vi "create junit report.vi"(8 "Error In (No Error)":errorcluster, 10 "junit report file path":path, 11 "test results":T3) -> (0 "Error Out":errorcluster)   [LabVIEW 2013]
uses:
  <vilib>/utf/dialogs/utf_testsuite_report_sortby.ctl
  <vilib>/utf/results/utf_report_summary.ctl
  <vilib>/utf/common/utf_test_result_overall.ctl
  <vilib>/utf/common/utf_test_result_testfile.ctl
  <vilib>/utf/common/utf_test_result_testcase.ctl
  <vilib>/utf/common/utf_test_result.ctl
  <vilib>/utf/common/utf_test_result_troll_new.ctl
  <vilib>/utf/common/utf_vector_result.ctl
  <vilib>/utf/common/utf_test_result_failure.ctl
  <vilib>/utf/common/utf_test_comparison_operators.ctl
  <vilib>/utf/common/utf_vi_tag.ctl
  <vilib>/utf/common/utf_test_result_input_data.ctl
  <vilib>/utf/common/utf_code_coverage.ctl
  <vilib>/utf/common/utf_error_data.ctl
  <vilib>/utf/common/utf_error_type.ctl
  <vilib>/utf/common/utf_subvi_info.ctl
  <vilib>/utf/dialogs/utf_testsuite_report_settings.ctl
  <vilib>/NI/JUnit Results API/Controls/Test Suites Attribute Values.ctl
  <vilib>/NI/JUnit Results API/Controls/Test Case Attributes.ctl
  <vilib>/NI/JUnit Results API/Controls/Outcome Attributes.ctl
  <vilib>/xml/Close Reference(Node).vi
  <vilib>/NI/JUnit Results API/JUnit API.lvlib
  <vilib>/xml/NI_XML.lvlib
  <vilib>/utf/NI_UnitTestFramework.lvlib
panel:
  in  "Report config":T1={"View Report ATML"=FALSE, "Create text report"=FALSE, "TEXT Sort by"=0, "ASCII report Path (*.txt)"=path "", "Create html report"=FALSE, "HTML report Path (*.html)"=path "", "Create atml report"=FALSE, "ATML report Path (*.xml)"=path "", "Summary Data"=FALSE, "Failed Tests"=TRUE, "Failed Tests Details"=TRUE, "Passed Tests"=TRUE, "Passed Tests Details"=TRUE, "Skipped Tests"=FALSE, "Errors"=FALSE, "Stylesheet file (*.css)"=path "", "Use stylesheet"=TRUE, "View Report HTML"=FALSE, "View Report TXT"=FALSE, "Errors Detail"=FALSE, "calculate project code coverage"=FALSE} {"TEXT Sort by" items=["VI name", "Test name"]}
  out "summary":T17
  in  "Sort by":T2=1 items=["VI name", "Test name"]
  # "Report Settings"
  # "Sort by"
  # "Report Content"
  # "HTML Stylesheet"
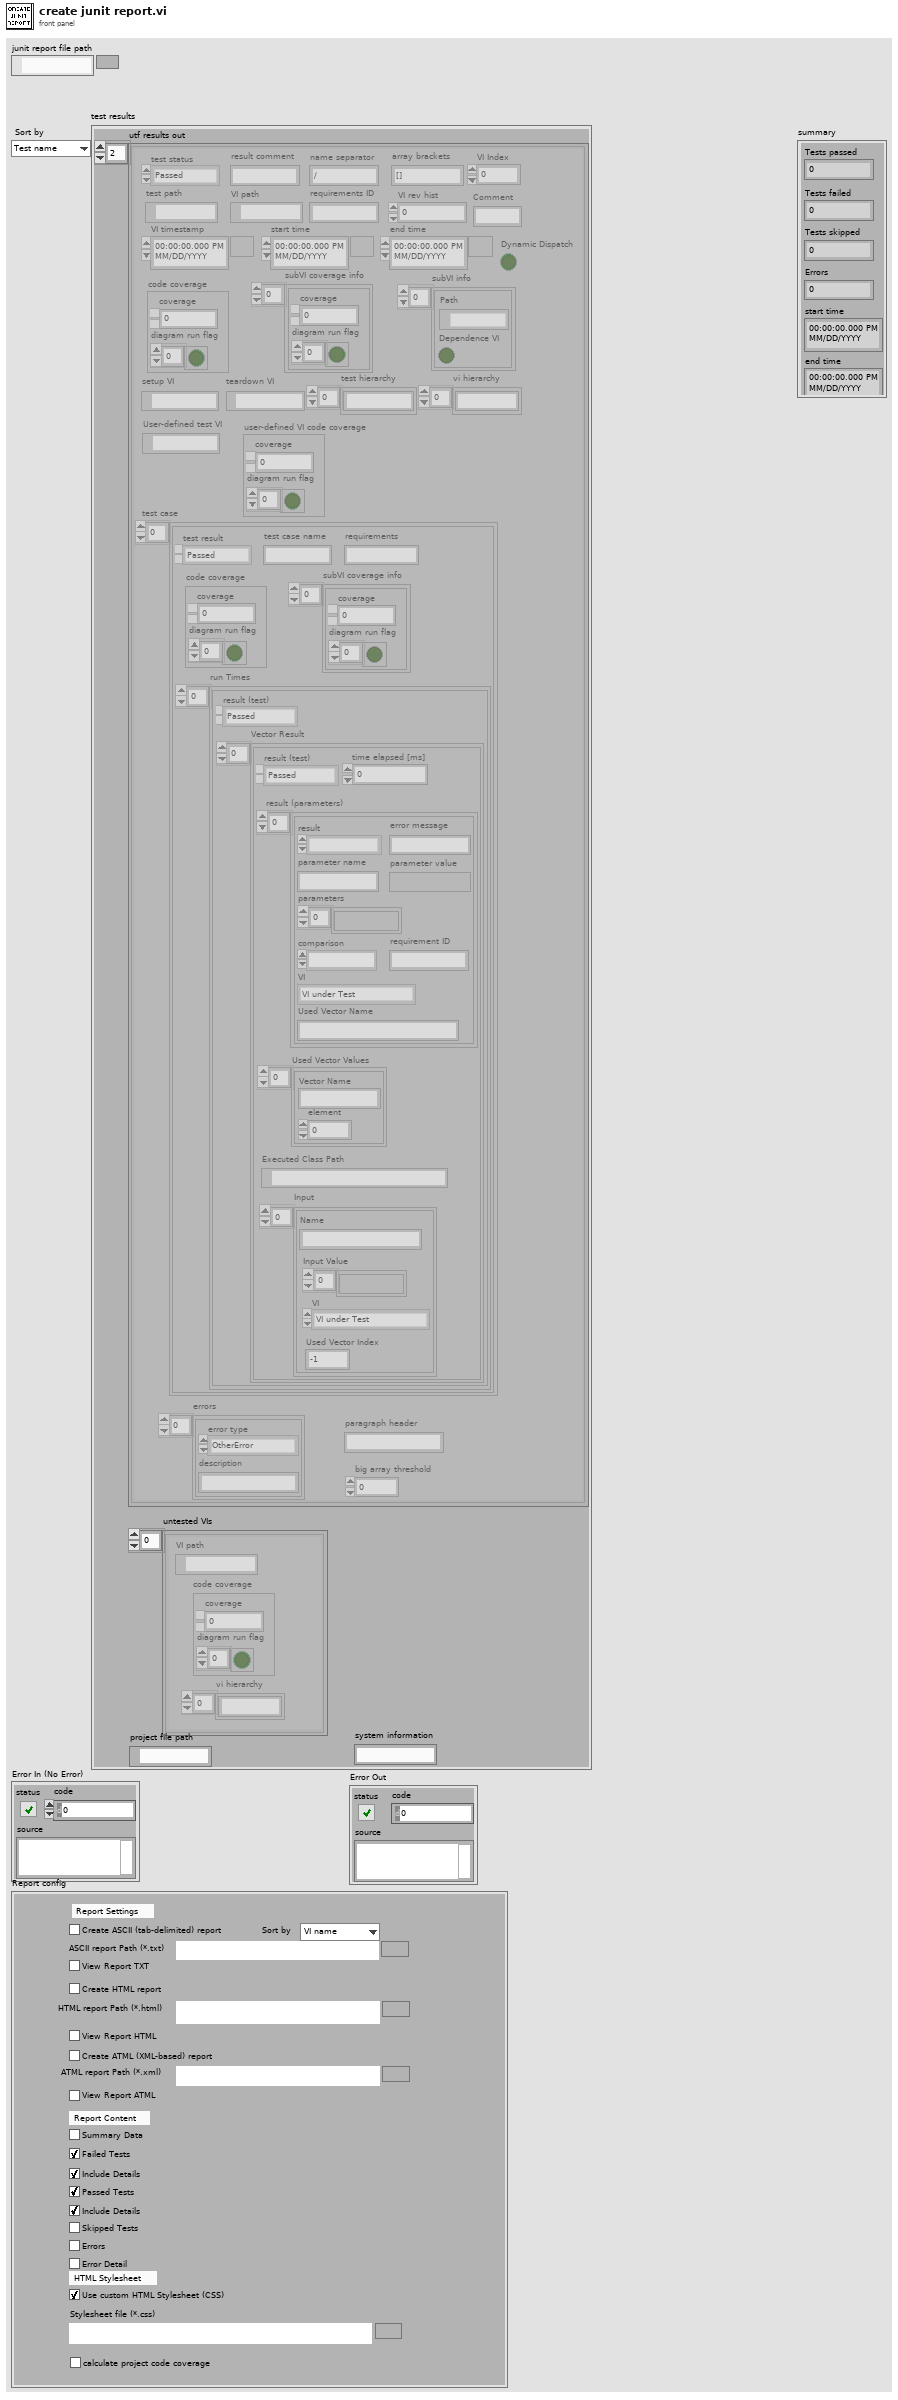
[diagram p1: front panel]
types:
  T1 = typedef "NI_UnitTestFramework.lvlib/utf_testsuite_report_settings.ctl" = cluster{"View Report ATML":bool, "Create text report":bool, "TEXT Sort by":T2, "ASCII report Path (*.txt)":path, "Create html report":bool, "HTML report Path (*.html)":path, "Create atml report":bool, "ATML report Path (*.xml)":path, "Summary Data":bool, "Failed Tests":bool, "Failed Tests Details":bool, "Passed Tests":bool, "Passed Tests Details":bool, "Skipped Tests":bool, "Errors":bool, "Stylesheet file (*.css)":path, "Use stylesheet":bool, "View Report HTML":bool, "View Report TXT":bool, "Errors Detail":bool, "calculate project code coverage":bool}
  T2 = typedef "NI_UnitTestFramework.lvlib/utf_testsuite_report_sortby.ctl" = u16
  T3 = typedef "NI_UnitTestFramework.lvlib/utf_test_result_overall.ctl" = cluster{"utf results out":T4[], "untested VIs":cluster{"VI path":path, "code coverage":T13, "vi hierarchy":string[]}[], "project file path":path, "system information":string}
  T4 = typedef "NI_UnitTestFramework.lvlib/utf_test_result_testfile.ctl" = cluster{"test case":T5[], "test status":T6, "test path":path, "setup VI":path, "teardown VI":path, "code coverage":T13, "start time":timestamp, "end time":timestamp, "test hierarchy":string[], "VI path":path, "VI timestamp":timestamp, "VI rev hist":i32, "requirements ID":string, "array brackets":string, "name separator":string, "errors":T14[], "paragraph header":string, "result comment":string, "vi hierarchy":string[], "subVI coverage info":T13[], "subVI info":T16[], "big array threshold":u32, "VI Index":i32, "Comment":string, "Dynamic Dispatch":bool, "User-defined test VI":path, "user-defined VI code coverage":T13}
  T5 = typedef "NI_UnitTestFramework.lvlib/utf_test_result_testcase.ctl" = cluster{"test result":T6, "run Times":T7[], "test case name":string, "requirements":string, "code coverage":T13, "subVI coverage info":T13[]}
  T6 = typedef "NI_UnitTestFramework.lvlib/utf_test_result.ctl" = enum16{"Passed", "Failed", "Error", "Skipped", "Not Processed"}
  T7 = typedef "NI_UnitTestFramework.lvlib/utf_test_result_troll_new.ctl" = cluster{"result (test)":T6, "Vector Result":T8[]}
  T8 = typedef "NI_UnitTestFramework.lvlib/utf_vector_result.ctl" = cluster{"time elapsed [ms]":u32, "result (test)":T6, "result (parameters)":T9[], "Used Vector Values":cluster{"Vector Name":string, "element":i32}[], "Executed Class Path":path, "Input":T12[]}
  T9 = typedef "NI_UnitTestFramework.lvlib/utf_test_result_failure.ctl" = cluster{"result":T6, "error message":string, "parameter name":string, "parameter value":variant, "parameters":variant[], "comparison":T10, "requirement ID":string, "VI":T11, "Used Vector Name":string}
  T10 = typedef "NI_UnitTestFramework.lvlib/utf_test_comparison_operators.ctl" = enum16{"=", "!=", ">", ">=", "<", "<=", "range", "symmetric tolerance", "asymmetric tolerance", "string contains", "string not contain", "array size", "string length", "array range", "by element", "array range (limit array)", "user-defined", "array contains", "array not contain", "vector length", "= (elm)", "!= (elm)", "= (case insensitive)", "!= (case insensitive)"}
  T11 = typedef "NI_UnitTestFramework.lvlib/utf_vi_tag.ctl" = enum16{"Setup VI", "VI under Test", "Teardown VI"}
  T12 = typedef "NI_UnitTestFramework.lvlib/utf_test_result_input_data.ctl" = cluster{"Name":string, "Input Value":variant[], "VI":T11, "Used Vector Index":i32}
  T13 = typedef "NI_UnitTestFramework.lvlib/utf_code_coverage.ctl" = cluster{"coverage":dbl, "diagram run flag":bool[]}
  T14 = typedef "NI_UnitTestFramework.lvlib/utf_error_data.ctl" = cluster{"error type":T15, "description":string}
  T15 = typedef "NI_UnitTestFramework.lvlib/utf_error_type.ctl" = enum16{"TestFileError", "VIError", "SetupVIError", "TearDownVIError", "OtherError"}
  T16 = typedef "NI_UnitTestFramework.lvlib/utf_subvi_info.ctl" = cluster{"Path":path, "Dependence VI":bool}
  T17 = typedef "NI_UnitTestFramework.lvlib/utf_report_summary.ctl" = cluster{"Tests passed":i32, "Tests failed":i32, "Tests skipped":i32, "Errors":i32, "start time":timestamp, "end time":timestamp}
  T18 = typedef "JUnit API.lvlib/Test Suites Attribute Values.ctl" = cluster{"name":string, "time":dbl, "tests":i32, "failures":i32, "disabled":i32, "errors":i32}
  T19 = typedef "JUnit API.lvlib/Test Case Attributes.ctl" = cluster{"name":string, "assertions":i32, "time":dbl, "timestamp":dbl, "classname":string, "status":string, "class":string, "file":string, "line":string, "log":string, "group":string, "url":string}
  T20 = typedef "JUnit API.lvlib/Outcome Attributes.ctl" = cluster{"message":string, "type":string}
  T21 = typedef "JUnit API.lvlib/Test Suite Attribute Values.ctl" = cluster{"name":string, "tests":i32, "failures":i32, "errors":i32, "time":dbl, "disabled":i32, "skipped":i32, "skips":i32, "timestamp":dbl, "hostname":string, "id":string, "package":string, "assertions":i32, "file":string, "skip":string, "log":string, "url":string}
  T22 = typedef "NI_UnitTestFramework.lvlib/utf_test_properties.ctl" = cluster{"Test File Header":T23, "Test Values":T27[], "Setup Teardown Info":T31, "Setup Values":T27[], "Teardown Values":T27[], "Vector Info":cluster{"included vector files":path[], "vector array":T34[], "included and inherited vector files":path[]}}
  T23 = typedef "NI_UnitTestFramework.lvlib/utf_test_file_header.ctl" = cluster{"Test Name":string, "Comment":string, "VI Under Test":path, "Library":path, "Priority":u32, "Test Vector Execution":T24, "Array Brackets":string, "Requirements ID":string, "Skip for project window":bool, "Skip for palette VI":bool, "Repetitions":u32, "Set time-out":bool, "Time-out":u32, "Check Code Coverage":bool, "Minimum Code Coverage":u32, "User-defined Test":bool, "Name Separator":string, "User-defined Test VI":path, "Precision":u8, "Creation Type":T25, "Decimal separator":string, "Big Array Threshold":u32, "Save control names in normal format":bool, "Capture Input Value":bool, "Capture Output Value":bool, "Version":string, "Set automatic error handling":T26, "Remove breakpoints":bool}
  T24 = typedef "NI_UnitTestFramework.lvlib/utf_test_processing.ctl" = enum16{"None", "Linear", "Permutations"}
  T25 = typedef "NI_UnitTestFramework.lvlib/utf_test_creation_type.ctl" = enum16{"Include controls and indicators from connector pane", "Include controls and indicators from front panel", "Include controls and indicators from front panel as both input and output"}
  T26 = typedef "NI_UnitTestFramework.lvlib/utf_set_automatic_error_handling.ctl" = enum16{"As is", "Enable", "Disable"}
  T27 = typedef "NI_UnitTestFramework.lvlib/utf_test_values_cluster.ctl" = cluster{"Input Values Array":T28[], "Expected Values Array":T30[], "Test Case Name":string, "Test Case Comment":string}
  T28 = typedef "NI_UnitTestFramework.lvlib/utf_test_input_values.ctl" = cluster{"Name":string, "Data type":T29, "Input Value":variant[], "Default Flag":bool, "Requirements ID":string, "Array Type":i8, "Typedef Flag":bool, "Setup Flag":bool, "Terminal":string, "Global Variable":bool, "type information":variant, "Shared Variable":bool, "Use Vector":bool, "Vector Name":string, "Index":u8}
  T29 = typedef "VariantType.lvlib/Type.ctl" = enum8{"Invalid Type", "Void", "I8", "I16", "I32", "I64", "U8", "U16", "U32", "U64", "Single Float", "Double Float", "Extended Float", "Single Complex", "Double Complex", "Extended Complex", "Enum U8", "Enum U16", "Enum U32", "Enum U64", "Single Float With Unit", "Double Float With Unit", "Extended Float With Unit", "Single Complex with Unit", "Double Complex with Unit", "Extended Complex with Unit", "Boolean", "String", "Path", "Picture", "Tag", "Array", "Cluster", "Variant", "LV Variant", "Waveform", "Timestamp", "Digital Waveform", "Digital Data", "ExpressData", "Refnum", "External Data", "VI", "Poly VI", "LabVIEW Class Instance", "Fixed Point"}
  T30 = typedef "NI_UnitTestFramework.lvlib/utf_test_expected_values.ctl" = cluster{"Name":string, "Data type":T29, "Expected value":variant, "Check flag":bool, "Typedef Flag":bool, "Comparison":T10, "User-defined Comparison VI":path, "Requirements ID":string, "Array Type":i8, "by element":dbl, "Teardown Flag":bool, "Terminal":string, "Global Variable":bool, "type information":variant, "Shared Variable":bool, "By Element":bool, "Use Vector":bool, "Vector Name":string}
  T31 = typedef "NI_UnitTestFramework.lvlib/utf_setup_teardown_info.ctl" = cluster{"Setup VI":path, "Teardown VI":path, "Setup Data":T32[], "Teardown Data":T33[]}
  T32 = typedef "NI_UnitTestFramework.lvlib/utf_setup_info.ctl" = cluster{"Terminal":string, "Input":string}
  T33 = typedef "NI_UnitTestFramework.lvlib/utf_teardown_info.ctl" = cluster{"Terminal":string, "Output":string}
  T34 = typedef "NI_UnitTestFramework.lvlib/utf_vector_info.ctl" = cluster{"requirement ID":string, "file path":path, "Data type":T29, "append":string, "size":u64, "name":string, "vector edit type":enum16{"sequence", "linear"}, "values":variant[], "qualify name":string}
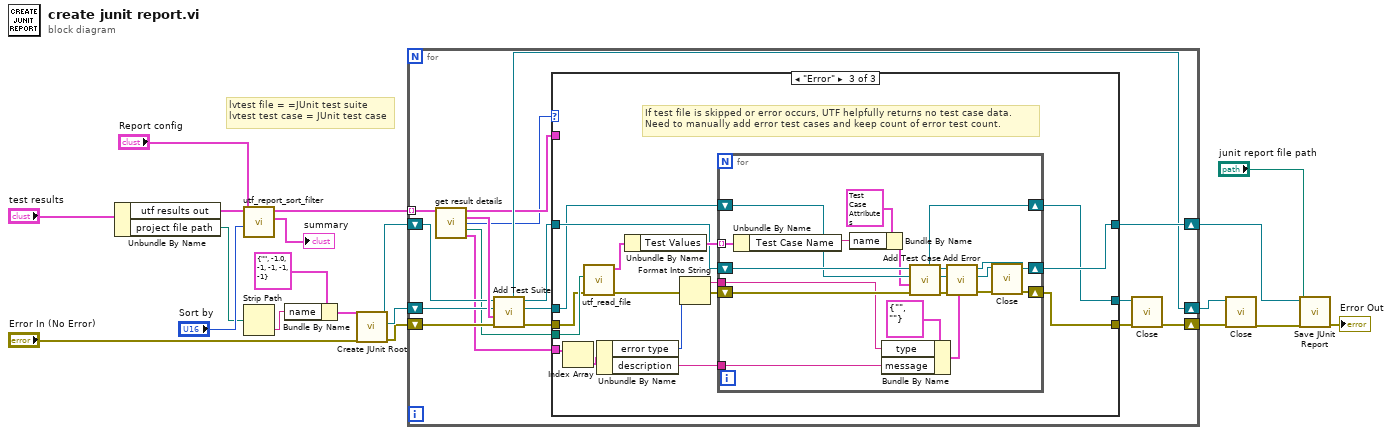
[diagram p0: block diagram]
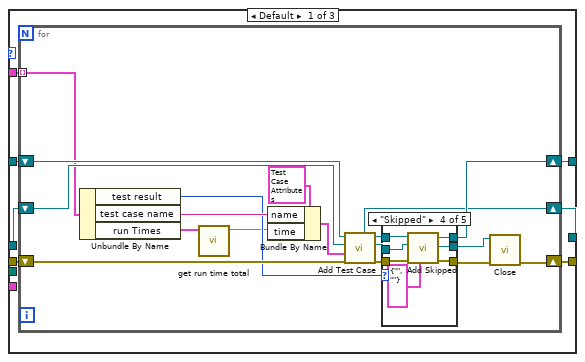
[diagram p2: hidden frame]
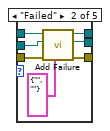
[diagram p4: hidden frame]
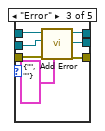
[diagram p5: hidden frame]
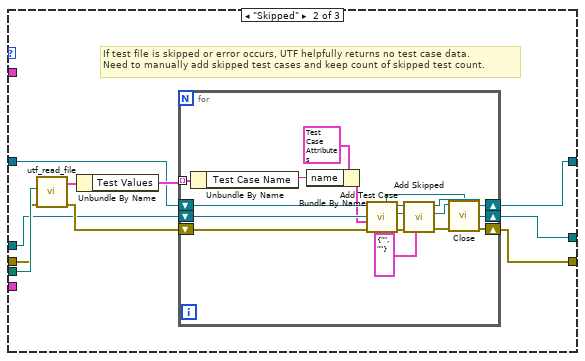
[diagram p7: hidden frame]
diagram:
  # "lvtest file = =JUnit test suite\nlvtest test case = JUnit test case"
  n1 = Unbundle By Name("test results") -> ("utf results out"=w20:T4[], "project file path"=w17:path)
  n2 = call <vilib>:"utf_report_sort_filter.vi"("Sort by"="Sort by", "Report config"="Report config", "test result"=w20) -> ("summary"=→"summary":T17, "test results filtered and sorted"=w16:T4[])  [unwired: 7 out]
  n3 = Strip Path(path=w17) -> (name=w7:string)  [unwired: 1 out]
  n4 = Bundle By Name(cluster=T18 {"name"="", "time"=-1.0, "tests"=-1, "failures"=-1, "disabled"=-1, "errors"=-1} ("Test Suites Atrributes"), "name"=w7) -> (w6:T18)
  n5 = call <vilib>:"Create JUnit Root.vi"("Error In (No Error)"="Error In (No Error)", "Test Suites Atrributes"=w6) -> ("Error Out"=w13:errorcluster, "Teststuites Ref"=w14:refnum<k20>, "File Ref Out"=w15:refnum<k20>)  [unwired: 7 in]
  n6 = for {
    tunnel: w16 -> [w37] mode=indexing
    shift-right: [w31] -> w12
    shift-left: w15 -> [w35]
    shift-right: [w28] -> w10
    shift-left: w14 -> [w34]
    shift-right: [w26] -> w9
    shift-left: w13 -> [w30]
    n7 = call "get result details.vi"("test result"=w37) -> ("test case"=w24:T5[], "Test Suites Atrributes"=w36:T21, "test status"=w23:T6, "test path"=w21:path, "errors"=w22:T14[])  [unwired: 10 in]
    n8 = call <vilib>:"Add Test Suite.vi"("Error In (No Error)"=w30, "Test Suite Atrributes"=w36, "Teststuites Ref In"=w34, "File Ref In"=w35) -> ("Error Out"=w29:errorcluster, "Testsuite Ref"=w32:refnum<k20>, "File Ref Out"=w33:refnum<k20>, "Teststuites Ref Out"=w28:refnum<k20>)  [unwired: 4 in]
    n9 = case shown="\"Error\"" w23 {
      tunnel: w33 -> [w44 w92 w125]
      tunnel: w32 -> [w43 w91 w124]
      tunnel: [w42 w93 w126] -> w31
      tunnel: w29 -> [w41 w96 w128]
      tunnel: [w40 w94 w127] -> w27
      tunnel: [w39 w90 w123] -> w25
      tunnel: w24 -> [w38 _ _]
      tunnel: w21 -> [_ w97 w129]
      tunnel: w22 -> [_ _ w122]
      frame Default {
        n10 = for {
          tunnel: w38 -> [w53] mode=indexing
          shift-right: [w57] -> w42
          shift-left: w44 -> [w61]
          shift-right: [w56] -> w39
          shift-left: w43 -> [w60]
          shift-right: [w48] -> w40
          shift-left: w41 -> [w55]
          n11 = Unbundle By Name(w53) -> ("test result"=w50:T6, "test case name"=w52:string, "run Times"=w46:T7[])
          n12 = call "get run time total.vi"("run Times"=w46) -> ("total time (ms)"=w45:dbl)  [unwired: 10 in]
          n13 = Bundle By Name(cluster=T19 {"name"="", "assertions"=0, "time"=0.0, "timestamp"=0.0, "classname"="", "status"="", "class"="", "file"="", "line"="", "log"="", "group"="", "url"=""} ("Test Case Atrributes"), "name"=w52, "time"=w45) -> (w51:T19)
          n14 = call <vilib>:"Add Test Case.vi"("Error In (No Error)"=w55, "Test Case Atrributes"=w51, "Testsuite Ref In"=w60, "File Ref In"=w61) -> ("error out"=w54:errorcluster, "Testcase Ref"=w58:refnum<k20>, "File Ref Out"=w59:refnum<k20>, "Testsuite Ref Out"=w56:refnum<k20>)  [unwired: 4 in]
          n15 = case shown="\"Skipped\"" w50 {
            tunnel: w59 -> [w65 w72 w78 w82 w88]
            tunnel: w58 -> [w63 w71 w77 w81 w89]
            tunnel: [w65 w70 w76 w83 w88] -> w57
            tunnel: w54 -> [w64 w69 w79 w86 w87]
            tunnel: [w64 w68 w74 w85 w87] -> w49
            tunnel: [w63 w67 w75 w84 w89] -> w47
            frame "Passed", Default {
            }
            frame "Failed" {
              n16 = call <vilib>:"Add Failure.vi"("Outcome Attributes"=T20 {"message"="", "type"=""}, "Error In (No Error)"=w69, "Testcase Ref"=w71, "File Ref In"=w72) -> ("Error Out"=w68:errorcluster, "Testcase Ref Out"=w67:refnum<k20>, "File Ref Out"=w70:refnum<k20>)  [unwired: 5 in]
            }
            frame "Error" {
              n17 = call <vilib>:"Add Error.vi"("Outcome Attributes"=T20 {"message"="", "type"=""}, "Error In (No Error)"=w79, "Testcase Ref"=w77, "File Ref In"=w78) -> ("Error Out"=w74:errorcluster, "Testcase Ref Out"=w75:refnum<k20>, "File Ref Out"=w76:refnum<k20>)  [unwired: 5 in]
            }
            frame "Skipped" {
              n18 = call <vilib>:"Add Skipped.vi"("Outcome Attributes"=T20 {"message"="", "type"=""}, "Error In (No Error)"=w86, "Testcase Ref"=w81, "File Ref In"=w82) -> ("Error Out"=w85:errorcluster, "Testcase Ref Out"=w84:refnum<k20>, "File Ref Out"=w83:refnum<k20>)  [unwired: 5 in]
            }
            frame "Not Processed" {
            }
          }
          n19 = call-poly <vilib>:"Close.vi"("error in (no error)"=w49, "node"=w47) -> ("error out"=w48:errorcluster)  [unwired: 7 in]
        }
      }
      frame "Skipped" {
        # "If test file is skipped or error occurs, UTF helpfully returns no test case data.\nNeed to manually add skipped test cases and keep count of skipped test count."
        n20 = call <vilib>:"utf_read_file.vi"("error in (no error)"=w96, "test file path"=w97) -> ("error out"=w95:errorcluster, "test specification out"=w98:T22)  [unwired: 5 in, 3 out]
        n21 = Unbundle By Name(w98) -> ("Test Values"=w99:T27[])
        n22 = for {
          tunnel: w99 -> [w115] mode=indexing
          shift-right: [w107] -> w94
          shift-left: w95 -> [w114]
          shift-right: [w102] -> w93
          shift-left: w92 -> [w110]
          shift-right: [w101] -> w90
          shift-left: w91 -> [w109]
          n23 = Unbundle By Name(w115) -> ("Test Case Name"=w105:string)
          n24 = Bundle By Name(cluster=T19 {"name"="", "assertions"=0, "time"=0.0, "timestamp"=0.0, "classname"="", "status"="", "class"="", "file"="", "line"="", "log"="", "group"="", "url"=""} ("Test Case Atrributes"), "name"=w105) -> (w104:T19)
          n25 = call <vilib>:"Add Test Case.vi"("Error In (No Error)"=w114, "Test Case Atrributes"=w104, "Testsuite Ref In"=w109, "File Ref In"=w110) -> ("error out"=w111:errorcluster, "Testcase Ref"=w112:refnum<k20>, "File Ref Out"=w113:refnum<k20>, "Testsuite Ref Out"=w101:refnum<k20>)  [unwired: 4 in]
          n26 = call <vilib>:"Add Skipped.vi"("Outcome Attributes"=T20 {"message"="", "type"=""}, "Error In (No Error)"=w111, "Testcase Ref"=w112, "File Ref In"=w113) -> ("Error Out"=w108:errorcluster, "Testcase Ref Out"=w103:refnum<k20>, "File Ref Out"=w102:refnum<k20>)  [unwired: 5 in]
          n27 = call-poly <vilib>:"Close.vi"("error in (no error)"=w108, "node"=w103) -> ("error out"=w107:errorcluster)  [unwired: 7 in]
        }
      }
      frame "Error" {
        # "If test file is skipped or error occurs, UTF helpfully returns no test case data.\nNeed to manually add error test cases and keep count of error test count."
        n28 = Index Array(array=w122) -> (element=w119:T14)  [unwired: 1 in]
        n29 = call <vilib>:"utf_read_file.vi"("error in (no error)"=w128, "test file path"=w129) -> ("error out"=w121:errorcluster, "test specification out"=w130:T22)  [unwired: 5 in, 3 out]
        n30 = Unbundle By Name(w119) -> ("error type"=w118:T15, "description"=w116:string)
        n31 = Unbundle By Name(w130) -> ("Test Values"=w131:T27[])
        n32 = Format Into String(error in=w121, w118) -> (resulting string=w117:string, error out=w120:errorcluster)  [unwired: 2 in]
        n33 = for {
          tunnel: w131 -> [w150] mode=indexing
          shift-right: [w142] -> w127
          shift-left: w120 -> [w149]
          shift-right: [w137] -> w126
          shift-left: w125 -> [w145]
          shift-right: [w136] -> w123
          shift-left: w124 -> [w144]
          tunnel: w117 -> [w133]
          tunnel: w116 -> [w132]
          n34 = Unbundle By Name(w150) -> ("Test Case Name"=w140:string)
          n35 = Bundle By Name(cluster=T19 {"name"="", "assertions"=0, "time"=0.0, "timestamp"=0.0, "classname"="", "status"="", "class"="", "file"="", "line"="", "log"="", "group"="", "url"=""} ("Test Case Atrributes"), "name"=w140) -> (w139:T19)
          n36 = Bundle By Name(cluster=T20 {"message"="", "type"=""} ("Outcome Attributes"), "type"=w133, "message"=w132) -> (w134:T20)
          n37 = call <vilib>:"Add Test Case.vi"("Error In (No Error)"=w149, "Test Case Atrributes"=w139, "Testsuite Ref In"=w144, "File Ref In"=w145) -> ("error out"=w146:errorcluster, "Testcase Ref"=w147:refnum<k20>, "File Ref Out"=w148:refnum<k20>, "Testsuite Ref Out"=w136:refnum<k20>)  [unwired: 4 in]
          n38 = call <vilib>:"Add Error.vi"("Outcome Attributes"=w134, "Error In (No Error)"=w146, "Testcase Ref"=w147, "File Ref In"=w148) -> ("Error Out"=w143:errorcluster, "Testcase Ref Out"=w138:refnum<k20>, "File Ref Out"=w137:refnum<k20>)  [unwired: 5 in]
          n39 = call-poly <vilib>:"Close.vi"("error in (no error)"=w143, "node"=w138) -> ("error out"=w142:errorcluster)  [unwired: 7 in]
        }
      }
    }
    n40 = call-poly <vilib>:"Close.vi"("error in (no error)"=w27, "node"=w25) -> ("error out"=w26:errorcluster)  [unwired: 7 in]
  }
  n41 = call-poly <vilib>:"Close.vi"("error in (no error)"=w9, "node"=w10) -> ("error out"=w11:errorcluster)  [unwired: 7 in]
  n42 = call <vilib>:"Save JUnit Report.vi"("Error In (No Error)"=w11, "XML file path"="junit report file path", "File Ref In"=w12) -> ("Error Out"=→"Error Out":errorcluster)  [unwired: 8 in]
